vi "Get Application.vi"(8 "error in (no error)":errorcluster, 11 "Test Class in":refnum<class "Test Class.lvclass">) -> (0 "error out":errorcluster, 2 "Application.lvlib:Application.lvclass":refnum<class "Application.lvclass">)   [LabVIEW 2017, in "Test Class.lvclass"]
uses:
  Test Class.lvclass
  Classes/Application/Class/Application.lvclass
  Test Class.lvclass/Test Class.ctl
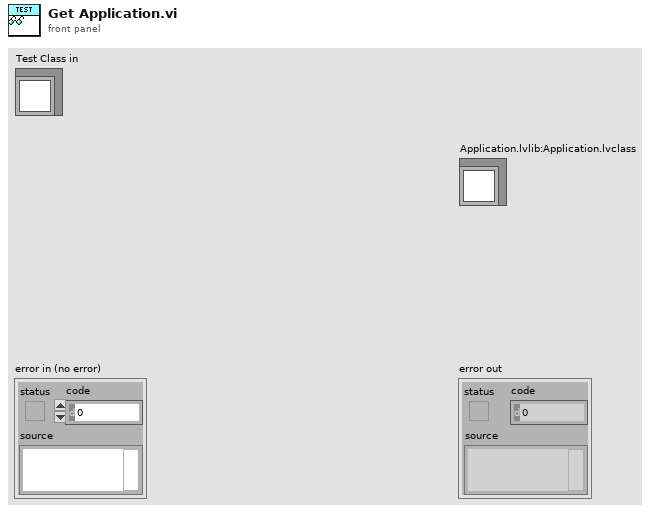
[diagram p1: front panel]
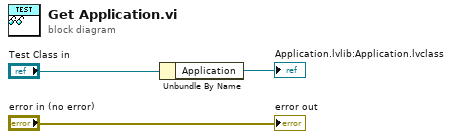
[diagram p0: block diagram]
diagram:
  n1 = Unbundle By Name("Test Class in") -> ("Application"=→"Application.lvlib:Application.lvclass":refnum<class "Application.lvclass">)
  "error out" <- "error in (no error)"
